vi "CRYStep Write.vi"(4 "StepIdentifier":string, 5 "Default":bool, 6 "Proper VI No":i32, 7 "Category Name":string, 8 "All/Name/Write(0,1,2)?":u8, 9 "Step File Path":path=path "C:/", 10 "Step flattened":string, 11 "Step File Name":string="Default Step.txt") -> (0 "File path":path, 1 "name":string, 3 "Cancel":bool)   [LabVIEW 2013]
uses:
  CRYProject/CRYProject Editor Global.vi
panel:
  out "Identfier(*.)":string
  out "Identfier(Regular Expression)":string
  in  "Symbol Index":i32
  in  "Down Step Name":string
  in  "Identfier":string
  out "UpLimit":i32
  out "DownLimit":i32
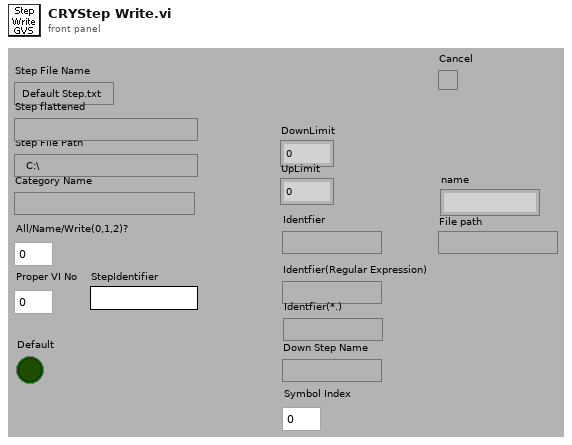
[diagram p1: front panel]
types:
  T1 = enum16{"OK", "Yes", "YesNo", "YesNoCancel", "ReplaceAppend"}
  T2 = enum16{"Left Button", "Center Button", "Right Button", "Window Close"}
  T3 = enum16{"open", "replace", "create", "open or create", "replace or create", "replace or create with confirmation"}
  T4 = cluster{"EventName":string, "Arg1":string, "Arg1 2":string, "Numeric":dbl, "Arg1 3":string}
  T5 = typedef "CRYStep.ctl" = cluster{"No.VI":i32, "Category":string, "StepName":string, "Seq setup flattened":string, "Comment":string, "Steps config.":bool[], "Jump config":i32[], "Start":dbl, "Increment":dbl, "Name":string, "Unit":string, "Y data":u16, "Y prefix":string, "Y dB ref":dbl, "Y unit":string, "Repeat State Array":cluster{"Start":dbl, "Increment":dbl, "Count":i32, "Num":i32}[]}
  T6 = enum16{"big-endian, network order", "native, host order", "little-endian"}
  T7 = typedef "CRYCalibration All Cluster.ctl" = cluster{"Calibration 2D":T8[], "Help":string, "Tab Value":i32, "Input Signal Type":string, "Output Signal Type":string}
  T8 = typedef "CRYCalibration 2DCluster.ctl" = cluster{"Calibration":T9, "Corr Curve":T10, "EQ Curve":T10, "Sens Curve":T10}
  T9 = typedef "CRYCalibration Cluster.ctl" = cluster{"Calibration Step Name":string, "Device":string, "Correction Curve Name":string, "Equalization Curve Name":string, "Sensitivity Curve Name":string, "Corr Folder and File":string, "EQ Folder and File":string, "Sens Folder and File":string, "Corr Step size":u16, "EQ Step size":u16, "Input":bool, "Last Cal Date (sec)":timestamp, "Cha Name":string, "Corr Curve Found":bool, "EQ Curve Found":bool, "Sens Curve Found":bool, "Signal Type":string, "Calibrated Device":string, "Hz":u32}
  T10 = typedef "CRYData Cluster.ctl" = cluster{"Name":string, "Curve":cluster{"x":dbl, "y":dbl, "z":dbl}[], "X data":u16, "Y data":u16, "Z data":u16, "X axis":u16, "Y axis":u16, "Z axis":u16, "X unit":string, "Y unit":string, "Z unit":string, "X dB ref":dbl, "Y dB ref":dbl, "Z dB ref":dbl, "single val":bool, "protected":bool, "display X":bool, "display Y":bool, "display Z":bool, "Test Info":string, "Step No.":i32, "Plot Settings":cluster{"Color":u32, "Interpolation":u8, "Point Style":u8, "Line Style":u8, "Point Color":u32, "Line Width":u8, "Bar Plot Style":u8, "Fill To":i16}, "AutoProtect":bool}
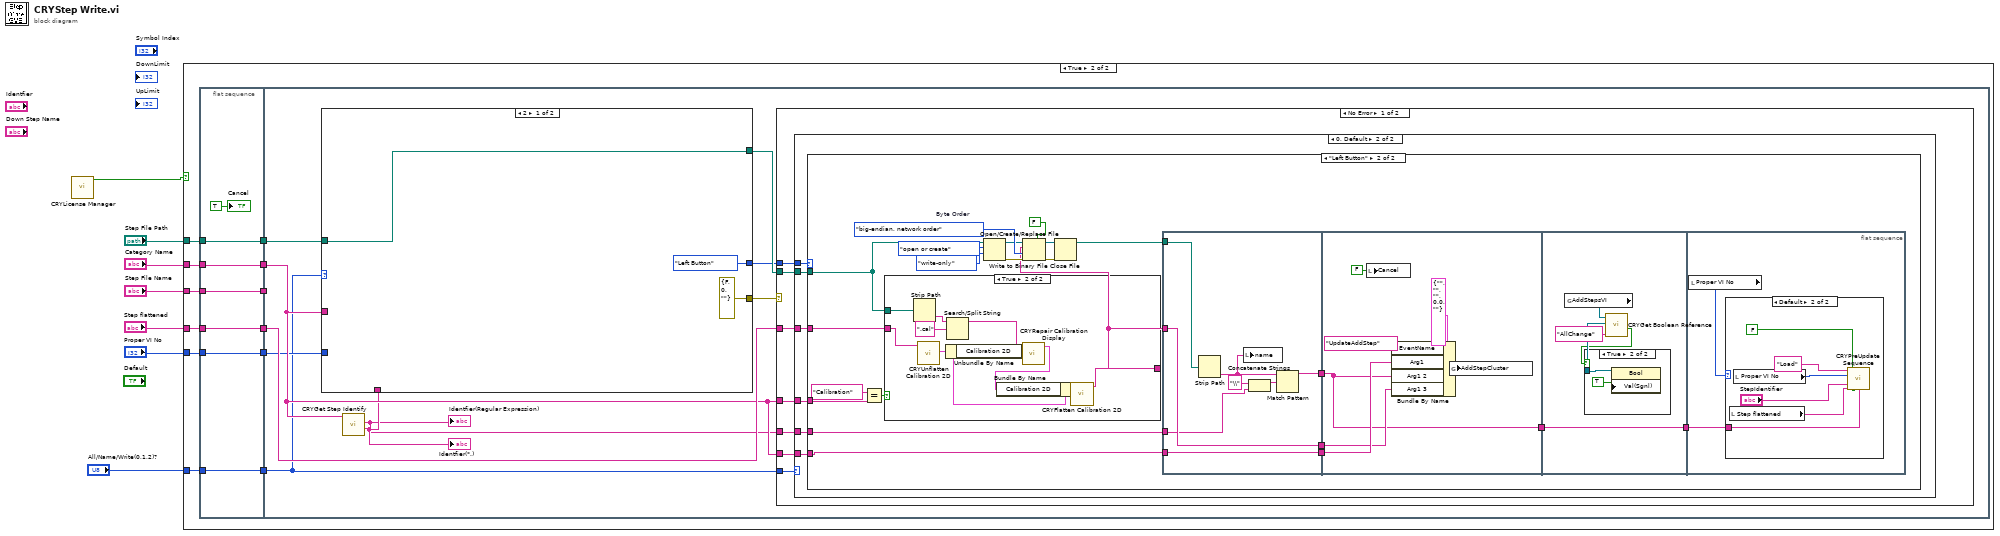
[diagram p0: block diagram]
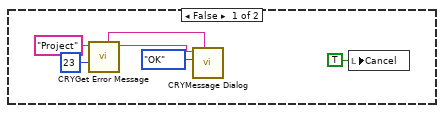
[diagram p2: hidden frame]
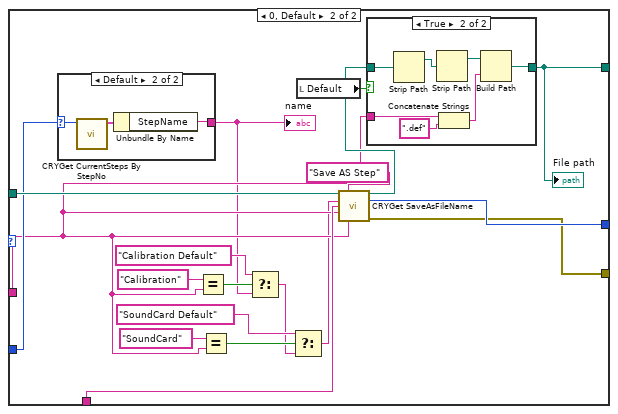
[diagram p3: hidden frame]
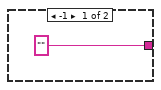
[diagram p4: hidden frame]
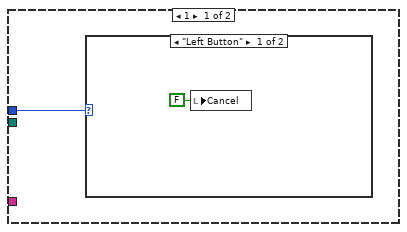
[diagram p6: hidden frame]
diagram:
  n1 = call "CRYLicense Manager.vi"() -> ("Test Result"=w2:bool)  [unwired: 10 in, 1 out]
  n2 = case shown="True" w2 {
    tunnel: "Step File Name" -> [_ w25]
    tunnel: "Step File Path" -> [_ w24]
    tunnel: "Step flattened" -> [_ w23]
    tunnel: "Category Name" -> [_ w22]
    tunnel: "Proper VI No" -> [_ w21]
    tunnel: "All/Name/Write(0,1,2)?" -> [_ w20]
    frame False {
      n3 = call "CRYGet Error Message.vi"("Error No"=23, "Kind"="Project") -> ("Message"=w13:string, "Window Title"=w9:string)  [unwired: 4 in, 4 out]
      n4 = call "CRYMessage Dialog.vi"("Window Title"=w9, "YesNoCancel"=T1."OK", "Message Content"=w13) -> ()  [unwired: 7 in, 2 out]
      n5 = local write "Cancel"(TRUE ("Cancel")) -> ()
    }
    frame True {
      n6 = flat-sequence {
        tunnel: w20 -> [w27]
        tunnel: w21 -> [w28]
        tunnel: w22 -> [w29]
        tunnel: w23 -> [w30]
        tunnel: w24 -> [w31]
        tunnel: w25 -> [w32]
        tunnel: [w32] -> w19
        tunnel: [w31] -> w18
        tunnel: [w30] -> w17
        tunnel: [w29] -> w16
        tunnel: [w28] -> w15
        tunnel: [w27] -> w14
        tunnel: w14 -> [w33]
        tunnel: w15 -> [w34]
        tunnel: w16 -> [w37]
        tunnel: w17 -> [w42]
        tunnel: w18 -> [w40]
        tunnel: w19 -> [_]
        frame #0 {
          "Cancel" <- TRUE ("Cancel")
        }
        frame #1 {
          n7 = call "CRYGet Step Identify.vi"("Category Name In"=w37) -> ("Identfier(*.)"=w36:string, "Identfier(Regular Expression)"=w35:string)  [unwired: 3 in, 6 out]
          "Identfier(*.)" <- w36
          "Identfier(Regular Expression)" <- w35
          n8 = case shown="2" w33 {
            tunnel: [w45 w63] -> w41
            tunnel: w37 -> [_ w49]
            tunnel: w40 -> [w45 w60]
            tunnel: [T2."Left Button" ("Which Button?") w59] -> w39
            tunnel: [errorcluster {"status"=FALSE, "code"=0, "source"=""} ("error out") w58] -> w38
            tunnel: w34 -> [_ w57]
            tunnel: w36 -> [_ w56]
            frame 2 {
            }
            frame 0, Default {
              n9 = case shown="Default" w57 {
                selector: w57 -> [_ w66]
                tunnel: ["" ("Original StepName") w68] -> w48
                frame -1 {
                }
                frame Default {
                  n10 = call "CRYGet CurrentSteps By StepNo.vi"("Step Setup VI No"=w66) -> ("Step"=w67:T5)  [unwired: 8 in, 2 out]
                  n11 = Unbundle By Name(w67) -> ("StepName"=w68:string)
                }
              }
              "name" <- w48
              n12 = Equal?(x="Calibration", y=w49) -> (x = y?=w54:bool)
              n13 = Equal?(x="SoundCard", y=w49) -> (x = y?=w51:bool)
              n14 = Select(t="Calibration Default" ("x"), s=w54, f=w48) -> (s? t:f=w47:string)
              n15 = Select(t="SoundCard Default" ("x"), s=w51, f=w47) -> (s? t:f=w46:string)
              n16 = local read "Default"() -> (w64:bool)
              n17 = call "CRYGet SaveAsFileName.vi"("Start path"=w60, "TitleName"="Save AS Step" ("prompt"), "default name"=w46, "pattern (all files)"=w56, "pattern label"=w49, "Category Name"=w49) -> ("Path"=w61:path, "Which Button?"=w59:T2, "error out"=w58:errorcluster)  [unwired: 3 in, 4 out]
              n18 = case shown="True" w64 {
                tunnel: w61 -> [w69 w76]
                tunnel: [w69 w73] -> w63
                tunnel: w49 -> [_ w71]
                frame False {
                }
                frame True {
                  n19 = Strip Path(path=w76) -> (stripped path=w75:path)  [unwired: 1 out]
                  n20 = Strip Path(path=w75) -> (stripped path=w74:path)  [unwired: 1 out]
                  n21 = Concatenate Strings(w71, ".def" ("string")) -> (w72:string)
                  n22 = Build Path(base path=w74, name or relative path=w72) -> (appended path=w73:path)
                }
              }
              "File path" <- w63
            }
          }
          n23 = case shown="No Error" w38 {
            tunnel: w42 -> [w83 _]
            tunnel: w41 -> [w82 _]
            tunnel: w37 -> [w81 _]
            tunnel: w39 -> [w80 _]
            tunnel: w35 -> [w79 _]
            tunnel: w37 -> [w78 _]
            tunnel: w33 -> [w77 _]
            frame No Error {
              n24 = case shown="0, Default" w77 {
                tunnel: w83 -> [_ w91]
                tunnel: w82 -> [_ w90]
                tunnel: w81 -> [_ w89]
                tunnel: w80 -> [w84 w88]
                tunnel: w79 -> [_ w87]
                tunnel: w78 -> [_ w86]
                frame 1 {
                  n25 = case shown="\"Left Button\"" w84 {
                    frame "Left Button" {
                      n26 = local write "Cancel"(FALSE ("Cancel")) -> ()
                    }
                    frame "Center Button", Default {
                    }
                  }
                }
                frame 0, Default {
                  n27 = case shown="\"Left Button\"" w88 {
                    tunnel: w90 -> [_ w93]
                    tunnel: w91 -> [_ w95]
                    tunnel: w89 -> [_ w113]
                    tunnel: w87 -> [_ w112]
                    tunnel: w86 -> [_ w98]
                    frame "Center Button", Default {
                    }
                    frame "Left Button" {
                      w107 = T6."big-endian, network order"  # Byte Order
                      n28 = Equal?(x="Calibration", y=w98) -> (x = y?=w96:bool)
                      n29 = case shown="True" w96 {
                        tunnel: w95 -> [w114 w124]
                        tunnel: [w114 w119] -> w94
                        tunnel: w93 -> [_ w116]
                        frame False {
                        }
                        frame True {
                          n30 = Strip Path(path=w116) -> (name=w117:string)  [unwired: 1 out]
                          n31 = call "CRYUnflatten Calibration 2D.vi"("Flattened Calibration"=w124) -> ("Calibration Step Out"=w122:T7)  [unwired: 8 in, 2 out]
                          n32 = Unbundle By Name(w122) -> ("Calibration 2D"=w123:T8[])
                          n33 = Search/Split String(string=w117, search string/char (-)=".cal") -> (substring before match=w115:string)  [unwired: 3 out]
                          n34 = call "CRYRepair Calibration Display.vi"("Calibration In"=w123, "Calibration Step Name"=w115) -> ("Calibration Out"=w121:T8[])  [unwired: 9 in]
                          n35 = Bundle By Name(cluster=w122, "Calibration 2D"=w121) -> (w120:T7)
                          n36 = call "CRYFlatten Calibration 2D.vi"("Calibration All Cluster"=w120) -> ("Calibration flattened"=w119:string)  [unwired: 10 in]
                        }
                      }
                      n37 = Open/Create/Replace File(file path (use dialog)=w93, operation (0:open)=T3."open or create", access (0:read/write)=enum16{"read/write", "read-only", "write-only"}."write-only") -> (refnum out=w104:refnum<file>, error out=w110:errorcluster)  [unwired: 1 in, 3 out]
                      n38 = Write to Binary File(file (use dialog)=w104, data=w94, error in=w110, 5:FALSE ("prepend array or string size? (T)"), 9:w107) -> (refnum out=w109:refnum<file>, error out=w111:errorcluster)  [unwired: 2 out]
                      n39 = Close File(refnum=w109, error in=w111) -> (path=w92:path)  [unwired: 1 out]
                      n40 = flat-sequence {
                        tunnel: w94 -> [w131]
                        tunnel: [w132] -> w103
                        tunnel: [w131] -> w102
                        tunnel: w113 -> [w130]
                        tunnel: [w130] -> w101
                        tunnel: w112 -> [w128]
                        tunnel: w92 -> [w125]
                        tunnel: w103 -> [w135]
                        tunnel: w102 -> [w136]
                        tunnel: w101 -> [w137]
                        tunnel: [w135] -> w100
                        tunnel: w100 -> [w144]
                        tunnel: [w144] -> w99
                        tunnel: w99 -> [w148]
                        frame #0 {
                          n41 = Strip Path(path=w125) -> (name=w126:string)  [unwired: 1 out]
                          n42 = local write "name"(w126) -> ()
                          n43 = Concatenate Strings("\\" ("string"), w128) -> (w127:string)
                          n44 = Match Pattern(string=w126, regular expression=w127) -> (before substring=w132:string)  [unwired: 4 out]
                        }
                        frame #1 {
                          n45 = local write "Cancel"(FALSE ("Cancel")) -> ()
                          n46 = Bundle By Name(cluster=T4 {"EventName"="", "Arg1"="", "Arg1 2"="", "Numeric"=0.0, "Arg1 3"=""} ("AddStepCluster"), "EventName"="UpdateAddStep", "Arg1"=w137, "Arg1 2"=w135, "Arg1 3"=w136) -> (w134:T4)
                          n47 = global write "CRYProject Editor Global.vi" "AddStepCluster"(w134) -> ()
                        }
                        frame #2 {
                          n48 = global read "CRYProject Editor Global.vi" "AddStepsVI"() -> (w140:refnum<vi>)
                          n49 = call "CRYGet Boolean Reference.vi"("Label Name"="AllChange", "VI Refnum"=w140) -> ("Exist?"=w142:bool, "Boolean Ref"=w143:refnum<vi>)  [unwired: 8 out]
                          n50 = case shown="True" w142 {
                            tunnel: w143 -> [_ w145]
                            frame False {
                            }
                            frame True {
                              n51 = property class="Bool"(reference=w145, "Val(Sgnl)"=TRUE) -> ()  [unwired: 1 in, 2 out]
                            }
                          }
                        }
                        frame #3 {
                          n52 = local read "Proper VI No"() -> (w147:i32)
                          n53 = case shown="Default" w147 {
                            tunnel: w148 -> [_ w154]
                            frame -1 {
                            }
                            frame Default {
                              n54 = local read "Step flattened"() -> (w153:string)
                              n55 = local read "Proper VI No"() -> (w152:i32)
                              n56 = call "CRYPreUpdate Sequence.vi"("EventName"="Load", "StepName Arg3"=w154, "Proper VI No"=w152, "Project View Step Name Identifier Arg1"="StepIdentifier", "Step flattened Arg2"=w153, "AllChangeFlg"=FALSE ("Name/Identifier")) -> ()  [unwired: 10 in]
                            }
                          }
                        }
                      }
                    }
                  }
                }
              }
            }
            frame Error {
            }
          }
        }
      }
    }
  }
